vi "Logging Settings Dialog.vi"(8 "error in (no error)":errorcluster, 11 "Settings in":T1 {"Voltage Limit" scale=0.0..155.0 scale format="%.3g"; "Hardware Configuration"."Baud Rate" items=["<0>"=0, "4800"=4800, "9600"=9600, "19200"=19200, "38400"=38400, "57600"=57600, "115200"=115200]}) -> (0 "error out":errorcluster, 1 "Cancelled?":bool, 2 "UI Refresh Needed?":bool, 3 "Settings out":T1 {"Voltage Limit" scale=0.0..155.0 scale format="%.3g"; "Hardware Configuration"."Baud Rate" items=["<0>"=0, "4800"=4800, "9600"=9600, "19200"=19200, "38400"=38400, "57600"=57600, "115200"=115200]})   [LabVIEW 2022 SP3, in "Settings.lvlib"]
doc: "Dialog for selecting user specified settings."
uses:
  Settings.lvlib
  Settings.ctl
  Acquisition/Hardware Configuration.ctl
  Logging/Logging Configuration.ctl
  Acquisition/Acquisition.lvlib
  Logging/Logging.lvlib
panel:
  in  "Sampling Interval (s)":dbl=1.0 min=0.015 max=60.0 step=0.01
  in  "Append File":bool
  in  "Enable Timestamp":bool
  in  "File Path":path
  in  "Log Interval (s)":dbl=1.0 min=0.015 max=60.0 step=0.01
  in  "Cancel":bool
  in  "OK Button":bool
  # "Non visible portion of dialog (needed for connector pane)."
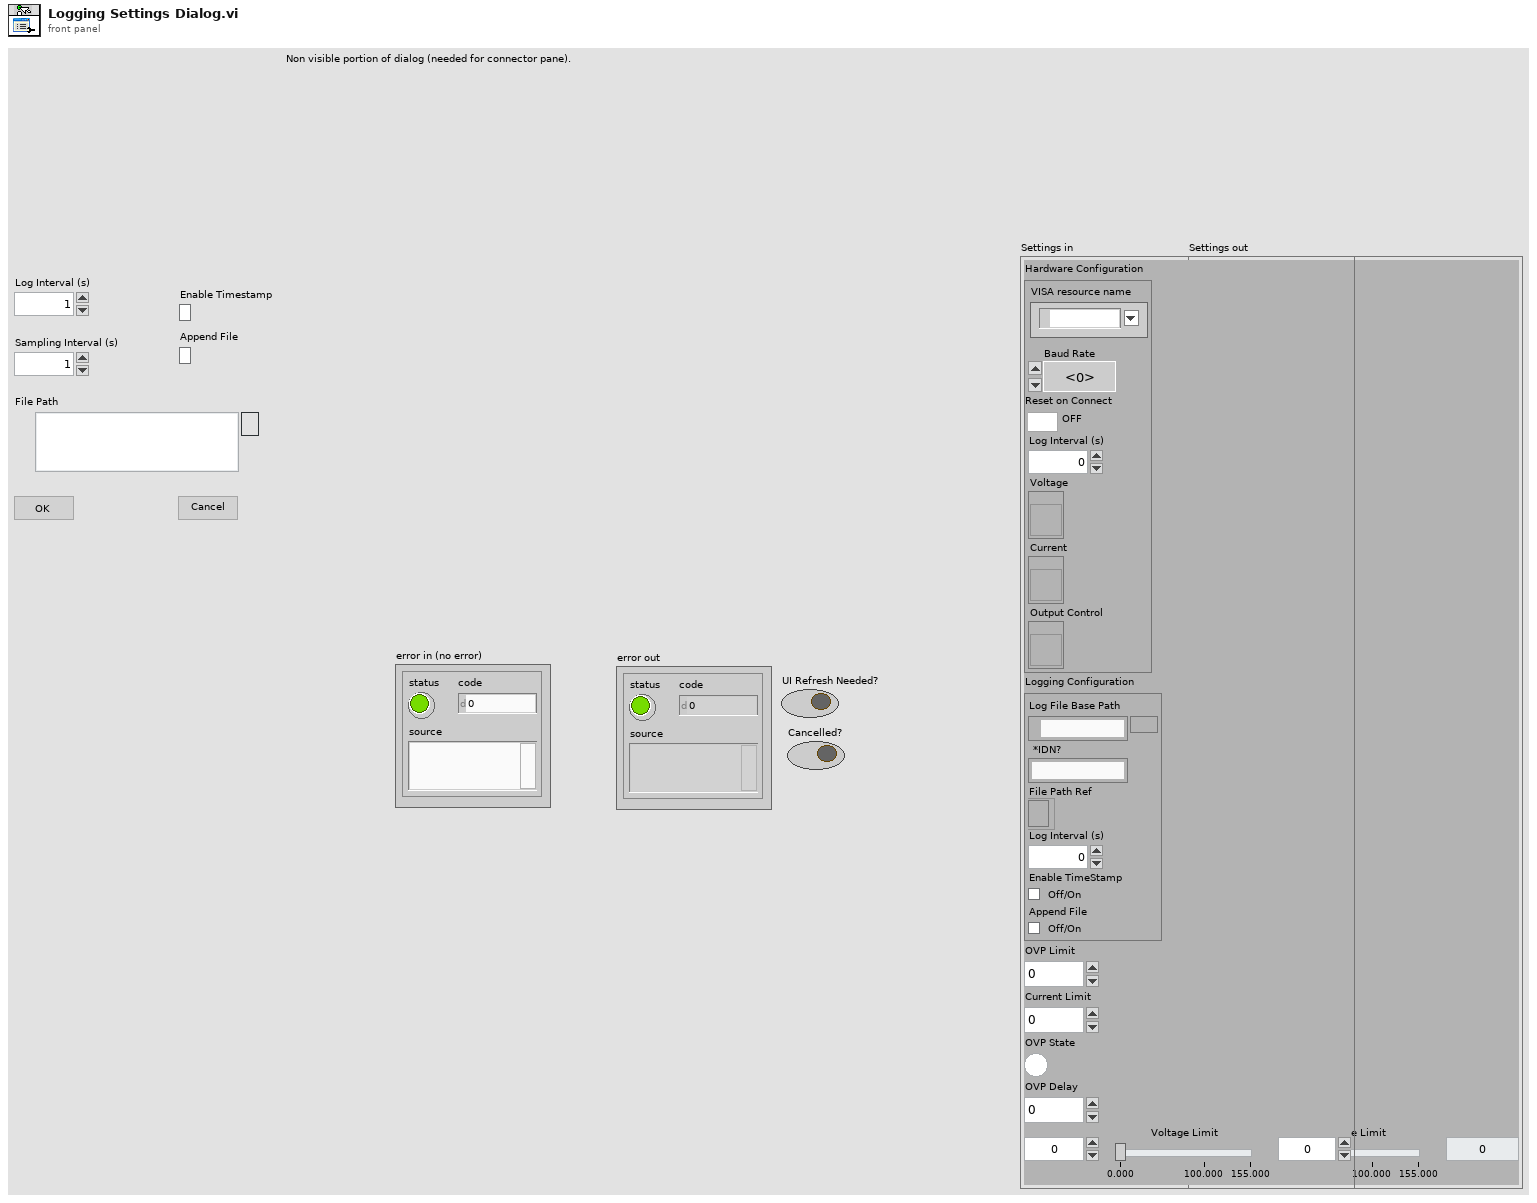
[diagram p1: front panel]
types:
  T1 = typedef "Settings.lvlib/Settings.ctl" = cluster{"Hardware Configuration":T2, "Logging Configuration":T3, "OVP Limit":dbl, "Current Limit":dbl, "OVP State":bool, "OVP Delay":dbl, "Voltage Limit":cluster{"Numeric":dbl, "Numeric":dbl}}
  T2 = typedef "Acquisition.lvlib/Hardware Configuration.ctl" = cluster{"VISA resource name":refnum<visa-resource-name>, "Baud Rate":u32, "Reset on Connect":bool, "Log Interval (s)":dbl, "Voltage":refnum<vi>, "Current":refnum<vi>, "Output Control":refnum<vi>}
  T3 = typedef "Logging.lvlib/Logging Configuration.ctl" = cluster{"Log File Base Path":path, "*IDN?":string, "File Path Ref":refnum<file>, "Log Interval (s)":dbl, "Enable TimeStamp":bool, "Append File":bool}
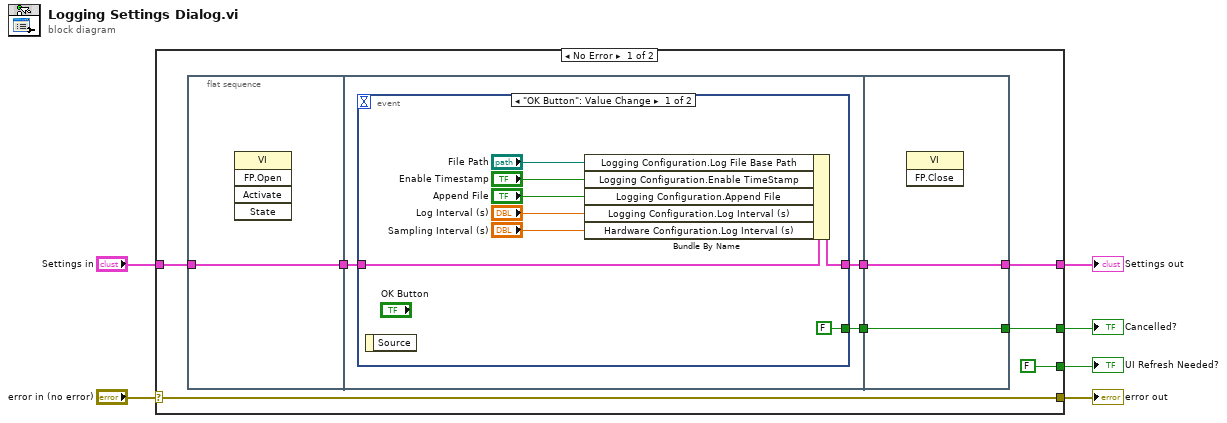
[diagram p0: block diagram]
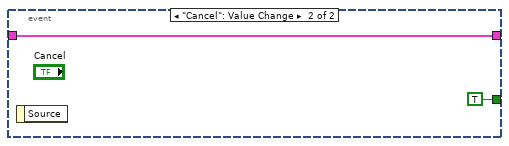
[diagram p2: hidden frame]
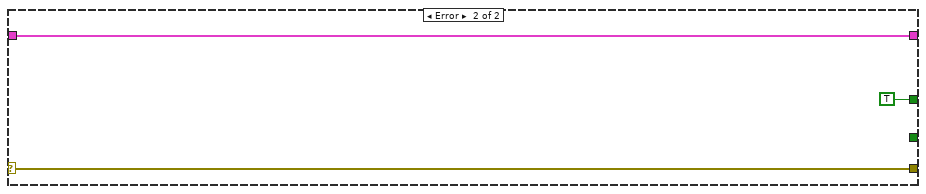
[diagram p3: hidden frame]
diagram:
  n1 = case shown="No Error" "error in (no error)" {
    selector: "error in (no error)" -> [w14 w33]
    tunnel: [w14 w33] -> w5
    tunnel: "Settings in" -> [w10 w32]
    tunnel: [w11 w32] -> w3
    tunnel: [FALSE ("UI Refresh Needed?") _] -> w2
    tunnel: [w12 TRUE ("UI Refresh Needed?")] -> w1
    frame No Error {
      n2 = flat-sequence {
        tunnel: w10 -> [w15]
        tunnel: [w15] -> w9
        tunnel: w9 -> [w16]
        tunnel: [w18] -> w8
        tunnel: [w17] -> w7
        tunnel: [w29] -> w11
        tunnel: [w30] -> w12
        tunnel: w8 -> [w30]
        tunnel: w7 -> [w29]
        frame #0 {
          n3 = invoke class="VI" method="FP.Open"() -> ()  [unwired: 5 in, 5 out]
        }
        frame #1 {
          n4 = event shown="[0] \"OK Button\": Value Change" {
            selector: _ -> [_ _]
            dyn-events: _ -> [_ _]
            timeout: _ -> [_ _]
            tunnel: [w24 w28] -> w17
            tunnel: w16 -> [w25 w28]
            tunnel: [FALSE ("UI Refresh Needed?") TRUE ("UI Refresh Needed?")] -> w18
            event "OK Button": Value Change {
              n5 = event-data() -> ()  [unwired: 1 in, 1 out]
              n6 = Bundle By Name(cluster=w25, "Logging Configuration.Log File Base Path"="File Path", "Logging Configuration.Enable TimeStamp"="Enable Timestamp", "Logging Configuration.Append File"="Append File", "Logging Configuration.Log Interval (s)"="Log Interval (s)", "Hardware Configuration.Log Interval (s)"="Sampling Interval (s)") -> (w24:T1)
            }
            event "Cancel": Value Change {
              n7 = event-data() -> ()  [unwired: 1 in, 1 out]
            }
          }
        }
        frame #2 {
          n8 = invoke class="VI" method="FP.Close"() -> ()  [unwired: 3 in, 3 out]
        }
      }
    }
    frame Error {
    }
  }
  "UI Refresh Needed?" <- w2
  "error out" <- w5
  "Settings out" <- w3
  "Cancelled?" <- w1
